vi "DAQ_Temp_Task.vi"(8 "error in":errorcluster) -> (0 "error out":errorcluster, 3 "task out":refnum<k21>)   [LabVIEW 2015]
uses:
  <vilib>/DAQmx/configure/timing.llb/DAQmx Timing (Sample Clock).vi
  <vilib>/DAQmx/create/channels.llb/DAQmx Create Channel (AI-Temperature-RTD).vi
  <vilib>/DAQmx/create/channels.llb/DAQmx Create Channel (TEDS-AI-Temperature-RTD).vi
  <resource>/objmgr/daqmx.rc
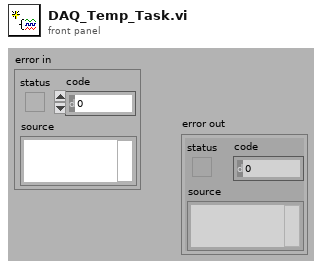
[diagram p1: front panel]
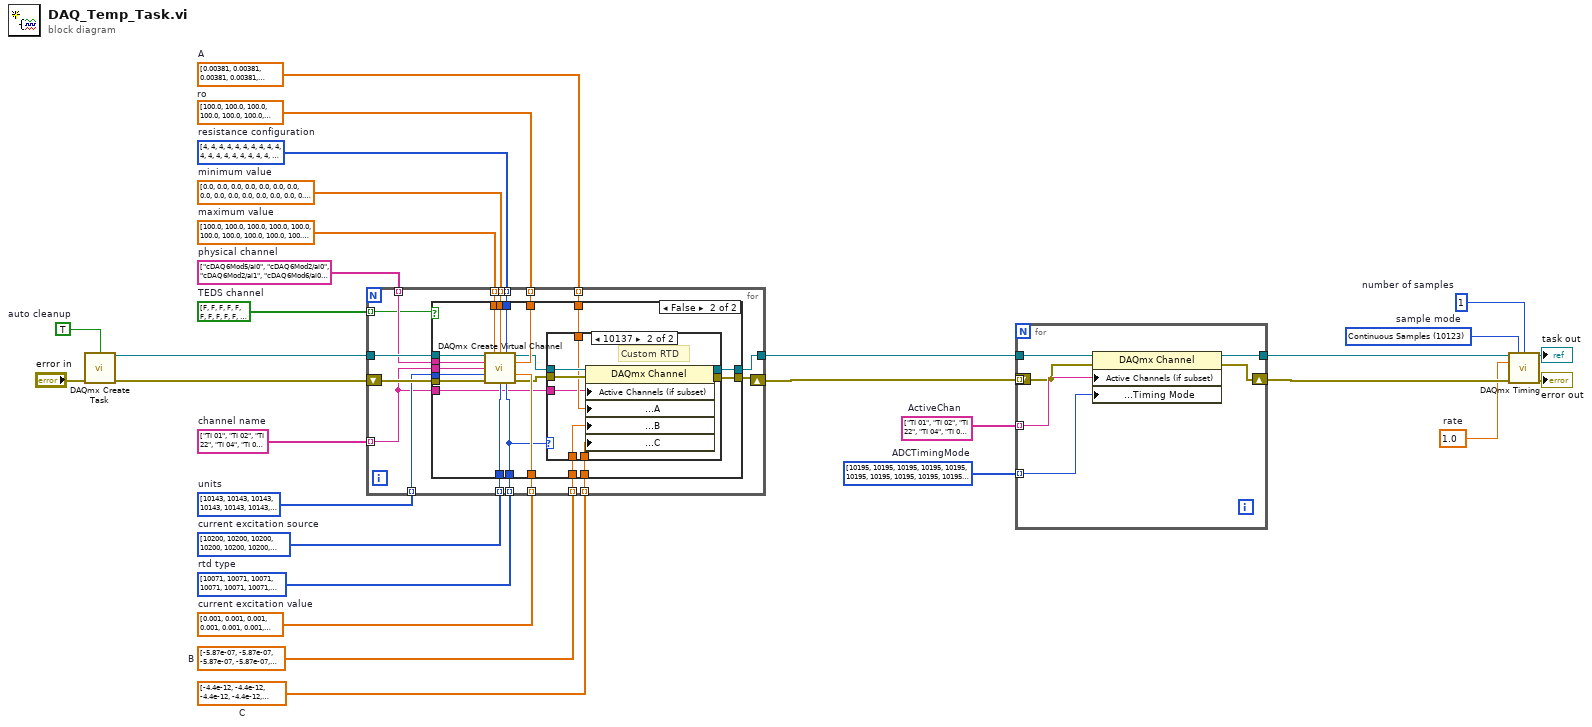
[diagram p0: block diagram]
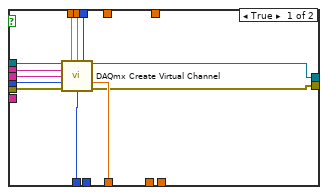
[diagram p2: hidden frame]
diagram:
  w1 = 10123 items=["Finite Samples"=10178, "Continuous Samples"=10123, "Hardware Timed Single Point"=12522]  # sample mode
  w2 = 1  # number of samples
  w3 = 1.0  # rate
  w8 = i32[] [10195, 10195, 10195, 10195, 10195, 10195, 10195, 10195, 10195, 10195, 10195, 10195, 10195, 10195, 10195, 10195, 10195, 10195, 10195, 10195, 10195, 10195, 10195, 10195, 10195, 10195, 10195, 10195] items=["High Resolution"=10195, "High Speed"=14712, "Best 50 Hz Rejection"=14713, "Best 60 Hz Rejection"=14714]  # ADCTimingMode
  w10 = string[] ["TI 01", "TI 02", "TI 22", "TI 04", "TI 05", "TI 06", "TI 06a", "TI 07", "TI 08", "TI 09", "TI 10", "TI 11", "TI 12", "TI 13", "TI 14", "TI 14a", "TI 20", "TI 21", "TI 21a", "TI 34", "TI 32", "TI 33", "TI 35", "TI 36", "TI 38", "TI 39", "Temp_Oelpruefstand", "TI 37"]  # ActiveChan
  w11 = bool[] [FALSE, FALSE, FALSE, FALSE, FALSE, FALSE, FALSE, FALSE, FALSE, FALSE, FALSE, FALSE, FALSE, FALSE, FALSE, FALSE, FALSE, FALSE, FALSE, FALSE, FALSE, FALSE, FALSE, FALSE, FALSE, FALSE, FALSE, FALSE]  # TEDS channel
  w12 = dbl[] [-4.4e-12, -4.4e-12, -4.4e-12, -4.4e-12, -4.4e-12, -4.4e-12, -4.4e-12, -4.4e-12, -4.4e-12, -4.4e-12, -4.4e-12, -4.4e-12, -4.4e-12, -4.4e-12, -4.4e-12, -4.4e-12, -4.4e-12, -4.4e-12, -4.4e-12, -4.4e-12, -4.4e-12, -4.4e-12, -4.4e-12, -4.4e-12, -4.4e-12, -4.4e-12, -4.4e-12, -4.4e-12]  # C
  w13 = dbl[] [-5.87e-07, -5.87e-07, -5.87e-07, -5.87e-07, -5.87e-07, -5.87e-07, -5.87e-07, -5.87e-07, -5.87e-07, -5.87e-07, -5.87e-07, -5.87e-07, -5.87e-07, -5.87e-07, -5.87e-07, -5.87e-07, -5.87e-07, -5.87e-07, -5.87e-07, -5.87e-07, -5.87e-07, -5.87e-07, -5.87e-07, -5.87e-07, -5.87e-07, -5.87e-07, -5.87e-07, -5.87e-07]  # B
  w14 = dbl[] [0.00381, 0.00381, 0.00381, 0.00381, 0.00381, 0.00381, 0.00381, 0.00381, 0.00381, 0.00381, 0.00381, 0.00381, 0.00381, 0.00381, 0.00381, 0.00381, 0.00381, 0.00381, 0.00381, 0.00381, 0.00381, 0.00381, 0.00381, 0.00381, 0.00381, 0.00381, 0.00381, 0.00381]  # A
  w17 = i32[] [10071, 10071, 10071, 10071, 10071, 10071, 10071, 10071, 10071, 10071, 10071, 10071, 10071, 10071, 10071, 10071, 10071, 10071, 10071, 10071, 10071, 10071, 10071, 10071, 10071, 10071, 10071, 10071] items=["Pt3750"=12481, "Pt3851"=10071, "Pt3911"=12482, "Pt3916"=10069, "Pt3920"=10053, "Pt3928"=12483, "Custom"=10137]  # rtd type
  w16 = dbl[] [0.001, 0.001, 0.001, 0.001, 0.001, 0.001, 0.001, 0.001, 0.001, 0.001, 0.001, 0.001, 0.001, 0.001, 0.001, 0.001, 0.001, 0.001, 0.001, 0.001, 0.001, 0.001, 0.001, 0.001, 0.001, 0.001, 0.001, 0.001]  # current excitation value
  w15 = dbl[] [100.0, 100.0, 100.0, 100.0, 100.0, 100.0, 100.0, 100.0, 100.0, 100.0, 100.0, 100.0, 100.0, 100.0, 100.0, 100.0, 100.0, 100.0, 100.0, 100.0, 100.0, 100.0, 100.0, 100.0, 100.0, 100.0, 100.0, 100.0]  # ro
  w22 = i32[] [10200, 10200, 10200, 10200, 10200, 10200, 10200, 10200, 10200, 10200, 10200, 10200, 10200, 10200, 10200, 10200, 10200, 10200, 10200, 10200, 10200, 10200, 10200, 10200, 10200, 10200, 10200, 10200] items=["Internal"=10200, "External"=10167, "None"=10230]  # current excitation source
  w21 = i32[] [10143, 10143, 10143, 10143, 10143, 10143, 10143, 10143, 10143, 10143, 10143, 10143, 10143, 10143, 10143, 10143, 10143, 10143, 10143, 10143, 10143, 10143, 10143, 10143, 10143, 10143, 10143, 10143] items=["deg C"=10143, "deg F"=10144, "Kelvins"=10325, "deg R"=10145, "From Custom Scale"=10065]  # units
  w20 = string[] ["TI 01", "TI 02", "TI 22", "TI 04", "TI 05", "TI 06", "TI 06a", "TI 07", "TI 08", "TI 09", "TI 10", "TI 11", "TI 12", "TI 13", "TI 14", "TI 14a", "TI 20", "TI 21", "TI 21a", "TI 34", "TI 32", "TI 33", "TI 35", "TI 36", "TI 38", "TI 39", "Temp_Oelpruefstand", "TI 37"]  # channel name
  w19 = string[] ["cDAQ6Mod5/ai0", "cDAQ6Mod2/ai0", "cDAQ6Mod2/ai1", "cDAQ6Mod6/ai0", "cDAQ6Mod1/ai0", "cDAQ6Mod1/ai1", "cDAQ6Mod3/ai1", "cDAQ6Mod3/ai0", "cDAQ6Mod4/ai1", "cDAQ6Mod4/ai0", "cDAQ6Mod7/ai0", "cDAQ6Mod6/ai2", "cDAQ6Mod6/ai3", "cDAQ6Mod3/ai2", "cDAQ6Mod3/ai3", "cDAQ6Mod6/ai1", "cDAQ6Mod5/ai3", "cDAQ6Mod5/ai1", "cDAQ6Mod5/ai2", "cDAQ6Mod7/ai1", "cDAQ6Mod2/ai2", "cDAQ6Mod2/ai3", "cDAQ6Mod1/ai2", "cDAQ6Mod1/ai3", "cDAQ6Mod4/ai3", "cDAQ6Mod4/ai2", "cDAQ6Mod7/ai2", "cDAQ6Mod7/ai3"]  # physical channel
  w23 = dbl[] [100.0, 100.0, 100.0, 100.0, 100.0, 100.0, 100.0, 100.0, 100.0, 100.0, 100.0, 100.0, 100.0, 100.0, 100.0, 100.0, 100.0, 100.0, 100.0, 100.0, 100.0, 100.0, 100.0, 100.0, 100.0, 100.0, 100.0, 100.0]  # maximum value
  w24 = dbl[] [0.0, 0.0, 0.0, 0.0, 0.0, 0.0, 0.0, 0.0, 0.0, 0.0, 0.0, 0.0, 0.0, 0.0, 0.0, 0.0, 0.0, 0.0, 0.0, 0.0, 0.0, 0.0, 0.0, 0.0, 0.0, 0.0, 0.0, 0.0]  # minimum value
  w25 = i32[] [4, 4, 4, 4, 4, 4, 4, 4, 4, 4, 4, 4, 4, 4, 4, 4, 4, 4, 4, 4, 4, 4, 4, 4, 4, 4, 3, 4] items=["2-Wire"=2, "3-Wire"=3, "4-Wire"=4]  # resistance configuration
  w27 = TRUE  # auto cleanup
  n1 = call <vilib>:"DAQmx Create Task.vi"("auto cleanup"=w27, "error in"="error in") -> ("task out"=w26:refnum<k21>, "error out"=w28:errorcluster)  [unwired: 12 in]
  n2 = for {
    tunnel: w26 -> [w44]
    tunnel: w25 -> [w45] mode=indexing
    tunnel: w24 -> [w46] mode=indexing
    tunnel: w23 -> [w47] mode=indexing
    tunnel: w22 -> [w40] mode=indexing
    tunnel: w21 -> [w41] mode=indexing
    tunnel: w20 -> [w30] mode=indexing
    tunnel: w19 -> [w42] mode=indexing
    tunnel: [w35] -> w7
    tunnel: w17 -> [w37] mode=indexing
    tunnel: w16 -> [w39] mode=indexing
    tunnel: w15 -> [w38] mode=indexing
    shift-right: [w36] -> w18
    shift-left: w28 -> [w43]
    tunnel: w14 -> [w34] mode=indexing
    tunnel: w13 -> [w33] mode=indexing
    tunnel: w12 -> [w32] mode=indexing
    tunnel: w11 -> [w31] mode=indexing
    n3 = case shown="False" w31 {
      tunnel: w47 -> [w59 w79]
      tunnel: w46 -> [w58 w78]
      tunnel: w45 -> [w57 w77]
      tunnel: w44 -> [w56 w76]
      tunnel: w43 -> [w55 w75]
      tunnel: w42 -> [w54 w74]
      tunnel: w41 -> [w53 w73]
      tunnel: w40 -> [w52 w72]
      tunnel: w39 -> [w51 w71]
      tunnel: w38 -> [_ w70]
      tunnel: w30 -> [w50 w69]
      tunnel: w37 -> [_ w68]
      tunnel: [w48 w65] -> w36
      tunnel: [w49 w64] -> w35
      tunnel: w34 -> [_ w63]
      tunnel: w33 -> [_ w62]
      tunnel: w32 -> [_ w61]
      tunnel: w30 -> [_ w60]
      frame True {
        n4 = call-poly <vilib>:"DAQmx Create Virtual Channel.vi"("task in"=w56, "maximum value"=w59, "minimum value"=w58, "resistance configuration"=w57, "physical channels"=w54, "name to assign"=w50, "units"=w53, "current excitation value"=w51, "error in"=w55, "current excitation source"=w52) -> ("task out"=w49:refnum<k21>, "error out"=w48:errorcluster)  [unwired: 4 in]
      }
      frame False {
        n5 = call-poly <vilib>:"DAQmx Create Virtual Channel.vi"("task in"=w76, "maximum value"=w79, "minimum value"=w78, "resistance configuration"=w77, "physical channels"=w74, "r0"=w70, "name to assign"=w69, "units"=w73, "current excitation value"=w71, "error in"=w75, "current excitation source"=w72, "rtd type"=w68) -> ("task out"=w67:refnum<k21>, "error out"=w66:errorcluster)  [unwired: 2 in]
        n6 = case shown="10137" w68 {
          tunnel: [w80 w89] -> w65
          tunnel: [w81 w88] -> w64
          tunnel: w67 -> [w81 w87]
          tunnel: w66 -> [w80 w86]
          tunnel: w63 -> [_ w83]
          tunnel: w62 -> [_ w85]
          tunnel: w61 -> [_ w84]
          tunnel: w60 -> [_ w82]
          frame 0, Default {
          }
          frame 10137 {
            # "Custom RTD"
            n7 = property class="DAQmx Channel"(reference=w87, error in=w86, "Active Channels (if subset)"=w82, "Analog Input:Temperature:RTD:Custom:A"=w83, "Analog Input:Temperature:RTD:Custom:B"=w85, "Analog Input:Temperature:RTD:Custom:C"=w84) -> (reference out=w88:refnum<k21>, error out=w89:errorcluster)
          }
        }
      }
    }
  }
  n8 = for {
    tunnel: w7 -> [w93]
    tunnel: w10 -> [w94] mode=indexing
    shift-right: [w95] -> w9
    shift-left: w18 -> [w91]
    tunnel: [w92] -> w4
    tunnel: w8 -> [w90] mode=indexing
    tunnel: [w91] -> _ mode=indexing
    n9 = property class="DAQmx Channel"(reference=w93, error in=w91, "Active Channels (if subset)"=w94, "Analog Input:General Properties:Digitizer/ADC:Timing Mode"=w90) -> (reference out=w92:refnum<k21>, error out=w95:errorcluster)
  }
  n10 = call-poly <vilib>:"DAQmx Timing.vi"("task/channels in"=w4, "sample mode"=w1, "samples per channel"=w2, "rate"=w3, "error in"=w9) -> ("task out"=→"task out":refnum<k21>, "error out"=→"error out":errorcluster)  [unwired: 9 in]
